vi "FPGA_VI.vi"() -> ()   [LabVIEW 2019]
uses:
  <vilib>/rvi/Emulation/niFpgaGetClockAttributes.vi
  <vilib>/rvi/Emulation/niFpgaSctlEmulationGetInTimedLoop.vi
  <vilib>/rvi/Emulation/niFpgaEmulationReportErrorSimple.vi
  <vilib>/rvi/eio/common/nirviEmuTemplateMethod_errors.vi
  <vilib>/rvi/Emulation/niFpgaCriticalErrorInLSC.vi
  <vilib>/eio/EIONode/EIONode.xnode
panel:
  in  "Wait (mSec)":u32
  in  "LED1":bool
  in  "LED0":bool
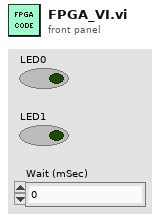
[diagram p1: front panel]
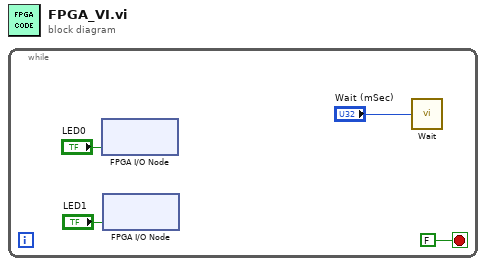
[diagram p0: block diagram]
diagram:
  n1 = while {
    stop <- FALSE stop-if-true
    n2 = xnode "FPGA I/O Node"("LED0"="LED0") -> ()  [unwired: 1 in, 1 out]
    n3 = xnode "FPGA I/O Node"("LED1"="LED1") -> ()  [unwired: 1 in, 1 out]
    n4 = call "Wait"("Count(mSec)"="Wait (mSec)") -> ()  [unwired: 1 out]
  }
